vi "Get NART Calibration Response From Response String.vi"(0 "Expected Response":T1, 5 "Response Subtype":T2, 7 "Expected Message start (\"\":any)":string, 9 "TCP Line":string, 11 "error in (no error)":errorcluster) -> (4 "NART Message":T3, 6 "More Pwr Reporting?":bool, 15 "error out":errorcluster)   [LabVIEW 2012]
uses:
  Controls/QCA NART Message.ctl
  Controls/QCA NART Response Type.ctl
  Controls/QCA NART Response SubType.ctl
  <vilib>/Utility/error.llb/whitespace.ctl
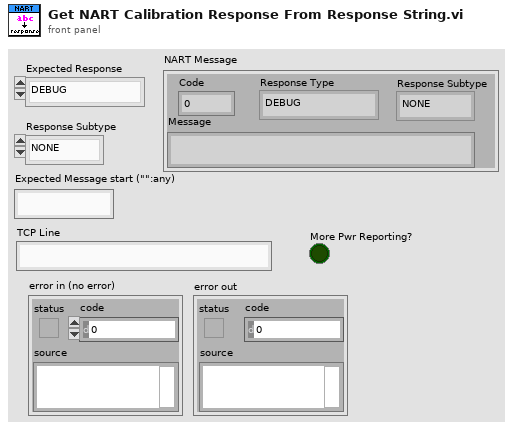
[diagram p1: front panel]
types:
  T1 = typedef "QCA NART Response Type.ctl" = enum16{"DEBUG", "CONTROL", "INFO", "WARNING", "ERROR", "NONE"}
  T2 = typedef "QCA NART Response SubType.ctl" = enum16{"NONE", "OK", "ON", "OFF", "BEGIN", "DONE"}
  T3 = typedef "QCA NART Message.ctl" = cluster{"Code":dbl, "Response Type":T1, "Response Subtype":T2, "Message":string}
  T4 = typedef "whitespace.ctl" = u16
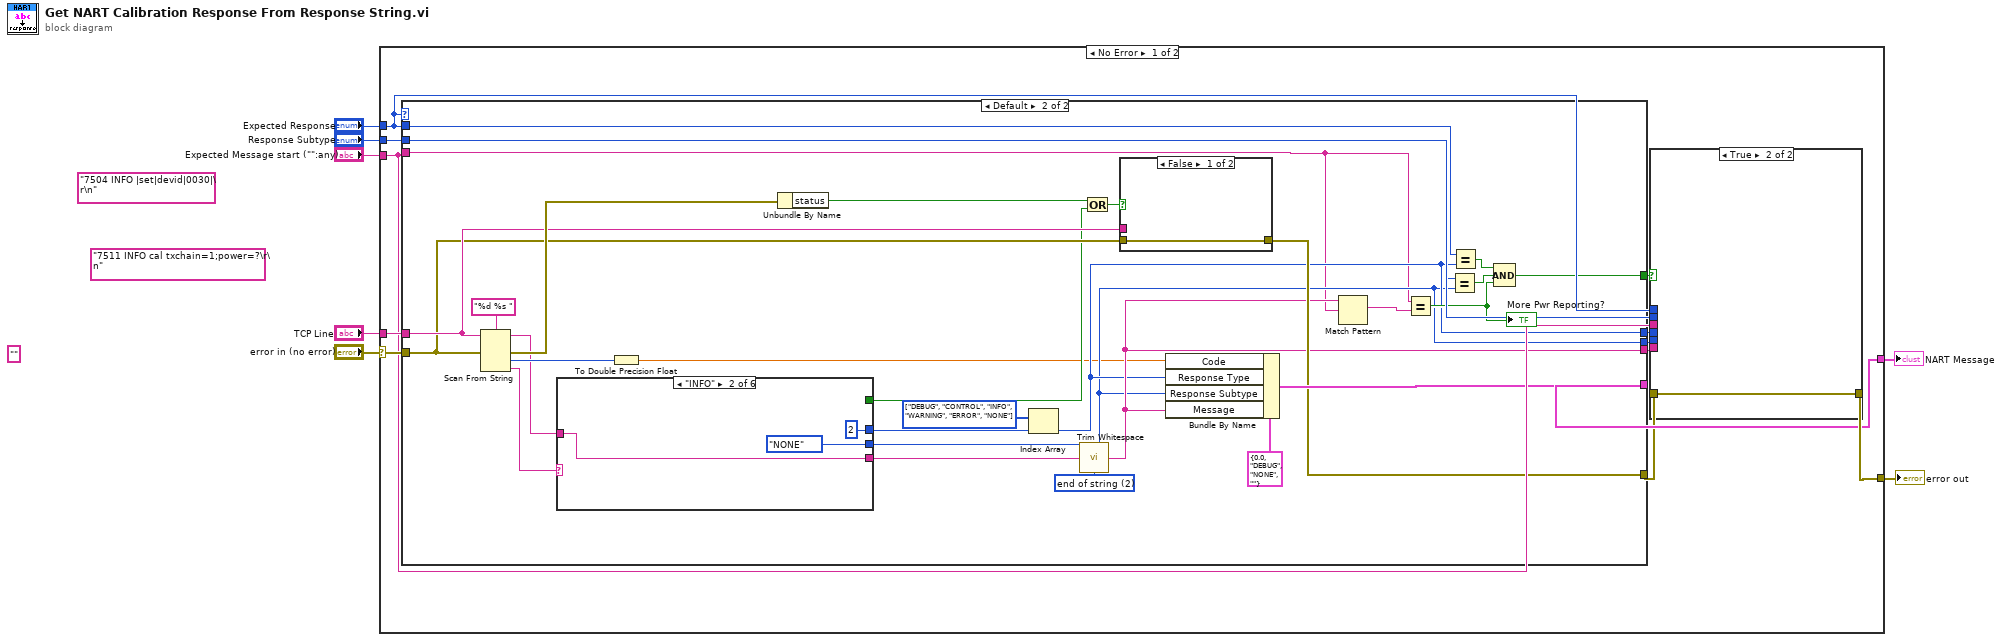
[diagram p0: block diagram]
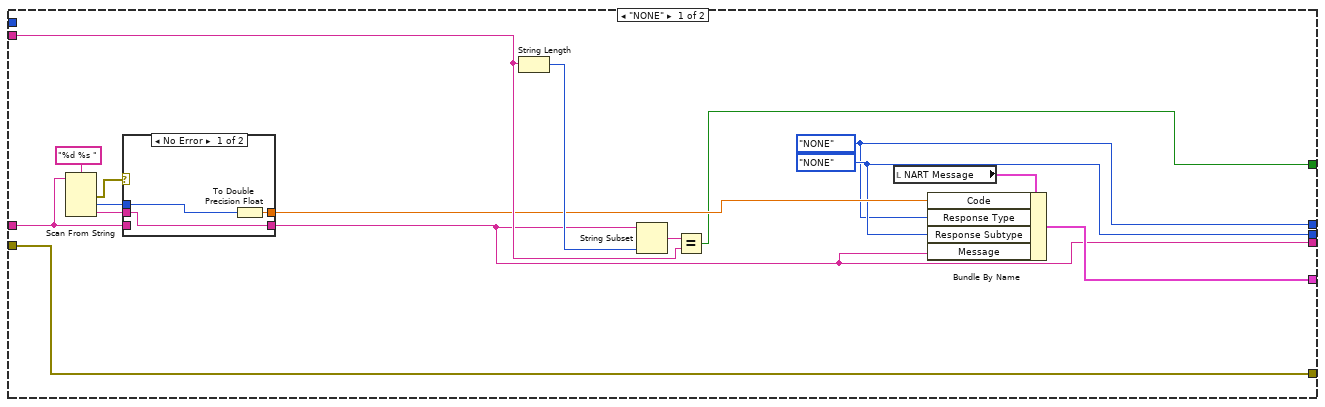
[diagram p2: hidden frame]
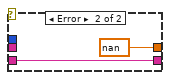
[diagram p3: hidden frame]
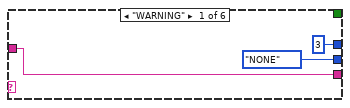
[diagram p4: hidden frame]
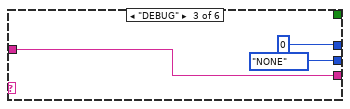
[diagram p5: hidden frame]
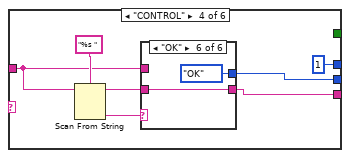
[diagram p6: hidden frame]
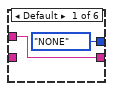
[diagram p7: hidden frame]
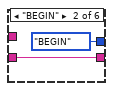
[diagram p8: hidden frame]
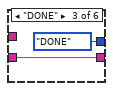
[diagram p9: hidden frame]
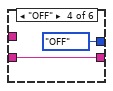
[diagram p10: hidden frame]
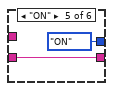
[diagram p11: hidden frame]
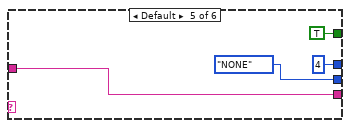
[diagram p12: hidden frame]
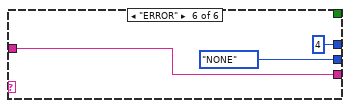
[diagram p13: hidden frame]
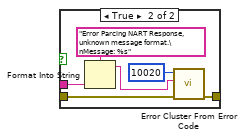
[diagram p14: hidden frame]
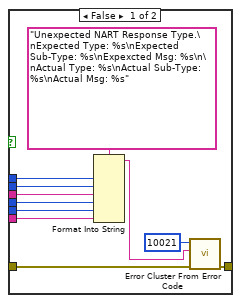
[diagram p15: hidden frame]
diagram:
  (unwired) ""
  (unwired) "7504 INFO |set|devid|0030|\r\n"
  (unwired) "7511 INFO cal txchain=1;power=?\r\n"
  n1 = case shown="No Error" "error in (no error)" {
    selector: "error in (no error)" -> [w11 w124]
    tunnel: [w19 w124] -> w7
    tunnel: [w18 _] -> w6
    tunnel: "Response Subtype" -> [w15 _]
    tunnel: "Expected Response" -> [w8 _]
    tunnel: "TCP Line" -> [w12 _]
    tunnel: "Expected Message start (\"\":any)" -> [w9 _]
    frame No Error {
      n2 = case shown="Default" w8 {
        tunnel: [w32 w69] -> w18
        tunnel: [w20 w49] -> w17
        tunnel: [w21 w43] -> w16
        tunnel: w15 -> [_ w68]
        tunnel: w8 -> [_ w67]
        tunnel: [w24 w66] -> w14
        tunnel: [w23 w57] -> w13
        tunnel: w12 -> [w22 w56]
        tunnel: w11 -> [w23 w55]
        tunnel: [w29 w52] -> w10
        tunnel: w9 -> [w34 w41]
        frame "NONE" {
          w20 = QCA_NART_Response_Type."NONE" ("Response Type")
          w21 = QCA_NART_Response_SubType."NONE" ("Response Subtype")
          n3 = Scan From String(format string="%d %s ", input string=w22) -> (error out=w27:errorcluster, output 1=w26:i32, output 2=w25:string)  [unwired: 4 in, 2 out]
          n4 = case shown="No Error" w27 {
            tunnel: w22 -> [_ w40]
            tunnel: [w38 nan ("Code")] -> w30
            tunnel: [w36 w40] -> w29
            tunnel: w26 -> [w37 _]
            tunnel: w25 -> [w36 _]
            frame No Error {
              n5 = To Double Precision Float(number=w37) -> (double precision float=w38:dbl)
            }
            frame Error {
            }
          }
          n6 = String Length(string=w34) -> (length=w33:i32)
          n7 = String Subset(string=w29, length (rest)=w33) -> (substring=w35:string)  [unwired: 1 in]
          n8 = Equal?(x=w35, y=w34) -> (x = y?=w24:bool)
          n9 = local read "NART Message"() -> (w31:T3)
          n10 = Bundle By Name(cluster=w31, "Code"=w30, "Response Type"=w20, "Response Subtype"=w21, "Message"=w29) -> (w32:T3)
        }
        frame Default {
          w50 = T1[] [enum."DEBUG", enum."CONTROL", enum."INFO", enum."WARNING", enum."ERROR", enum."NONE"] items=["DEBUG", "CONTROL", "INFO", "WARNING", "ERROR", "NONE"]
          w54 = T4 2 items=["both", "start of string", "end of string"] ("location (both)")
          n11 = Scan From String(format string="%d %s ", input string=w56, error in=w55) -> (remaining string=w45:string, error out=w62:errorcluster, output 1=w61:i32, output 2=w48:string)  [unwired: 3 in, 1 out]
          n12 = case shown="\"INFO\"" w48 {
            tunnel: [3 2 0 1 4 4] -> w47
            tunnel: [_ _ _ _ TRUE _] -> w46
            tunnel: w45 -> [w71 w74 w77 w81 w99 w102]
            tunnel: [w71 w74 w77 w79 w99 w102] -> w44
            tunnel: [QCA_NART_Response_SubType."NONE" ("Response Subtype") QCA_NART_Response_SubType."NONE" ("Response Subtype") QCA_NART_Response_SubType."NONE" ("Response Subtype") w80 QCA_NART_Response_SubType."NONE" ("Response Subtype") QCA_NART_Response_SubType."NONE" ("Response Subtype")] -> w43
            frame "WARNING" {
            }
            frame "INFO" {
            }
            frame "DEBUG" {
            }
            frame "CONTROL" {
              n13 = Scan From String(format string="%s ", input string=w81) -> (remaining string=w84:string, output 1=w83:string)  [unwired: 3 in, 2 out]
              n14 = case shown="\"OK\"" w83 {
                tunnel: w84 -> [_ w88 w90 w92 w94 w96]
                tunnel: w81 -> [w87 _ _ _ _ _]
                tunnel: [w87 w88 w90 w92 w94 w96] -> w79
                tunnel: [QCA_NART_Response_SubType."NONE" ("Response Subtype") QCA_NART_Response_SubType."BEGIN" ("Response Subtype") QCA_NART_Response_SubType."DONE" ("Response Subtype") QCA_NART_Response_SubType."OFF" ("Response Subtype") QCA_NART_Response_SubType."ON" ("Response Subtype") QCA_NART_Response_SubType."OK" ("Response Subtype")] -> w80
                frame Default {
                }
                frame "BEGIN" {
                }
                frame "DONE" {
                }
                frame "OFF" {
                }
                frame "ON" {
                }
                frame "OK" {
                }
              }
            }
            frame Default {
            }
            frame "ERROR" {
            }
          }
          n15 = To Double Precision Float(number=w61) -> (double precision float=w42:dbl)
          n16 = Unbundle By Name(w62) -> ("status"=w63:bool)
          n17 = Index Array(array=w50, index=w47) -> (element=w49:T1)
          n18 = call <vilib>:"Trim Whitespace.vi"("string"=w44, "location (both)"=w54) -> ("trimmed string"=w52:string)
          n19 = Or(x=w63, y=w46) -> (x .or. y?=w58:bool)
          n20 = case shown="False" w58 {
            tunnel: [w105 w108] -> w57
            tunnel: w56 -> [_ w107]
            tunnel: w55 -> [w105 w106]
            frame False {
            }
            frame True {
              n21 = Format Into String(format string="Error Parcing NART Response, unknown message format.\nMessage: %s", w107) -> (resulting string=w111:string)  [unwired: 2 in, 1 out]
              n22 = call <vilib>:"Error Cluster From Error Code.vi"("error in (no error)"=w106, "error message (\"\")"=w111, "error code (0)"=10020) -> ("error out"=w108:errorcluster)  [unwired: 6 in]
            }
          }
          n23 = Bundle By Name(cluster=T3 {"Code"=0.0, "Response Type"=enum."DEBUG", "Response Subtype"=enum."NONE", "Message"=""} ("NART Message"), "Code"=w42, "Response Type"=w49, "Response Subtype"=w43, "Message"=w52) -> (w69:T3)
          n24 = Match Pattern(string=w52, regular expression=w41) -> (match substring=w53:string)  [unwired: 1 in, 3 out]
          n25 = Equal?(x=w41, y=w53) -> (x = y?=w51:bool)
          "More Pwr Reporting?" <- w51
          n26 = Equal?(x=w68, y=w43) -> (x = y?=w65:bool)
          n27 = Equal?(x=w67, y=w49) -> (x = y?=w64:bool)
          n28 = Compound Arithmetic op=AND(w64, w65, w51) -> (w66:bool)
        }
      }
      n29 = case shown="True" w14 {
        tunnel: w13 -> [w122 w123]
        tunnel: [w114 w123] -> w19
        tunnel: w8 -> [w118 _]
        tunnel: w15 -> [w117 _]
        tunnel: w16 -> [w116 _]
        tunnel: w17 -> [w115 _]
        tunnel: w9 -> [w113 _]
        tunnel: w10 -> [w112 _]
        frame False {
          n30 = Format Into String(format string="Unexpected NART Response Type.\nExpected Type: %s\nExpected Sub-Type: %s\nExpexcted Msg: %s\n\nActual Type: %s\nActual Sub-Type: %s\nActual Msg: %s", w118, w117, w113, w115, w116, w112) -> (resulting string=w119:string)  [unwired: 2 in, 1 out]
          n31 = call <vilib>:"Error Cluster From Error Code.vi"("error in (no error)"=w122, "error message (\"\")"=w119, "error code (0)"=10021) -> ("error out"=w114:errorcluster)  [unwired: 6 in]
        }
        frame True {
        }
      }
    }
    frame Error {
    }
  }
  "error out" <- w7
  "NART Message" <- w6
